vi "ni579x Host Driven Synchronization.vi"(0 "Register Buses":T1[](array[typedef]), 11 "error in":errorcluster, 12 "sync.cptr.period":u16=13) -> (4 "Register Buses (out)":T1[](array[typedef]), 15 "error out":errorcluster)   [LabVIEW 2015, in "ni579x Synchronization v2 Host.lvlib"]
doc: "Use this flavor of synchronization in conjunction with \"ni579x Host Align\" on the FPGA. Please refer to the FPGA VIs for documentation. After this VI finishes, the FPGAs will be synchronized.\n\n<B>Input Parameters</B>\n\n<B>Register Buses</B> specifies the Register Buses to which the Synchronization library is connected in the FPGA VIs.\n\n<B>sync.cptr.period</B> is the period (in clocks) of the Common Periodic Time Reference (CPTR). The CPTR period controls the rate at which synchronized signals are realized. This parameter is optional, and defaults to 13.\n\nWhen using 'ni579x FPGA Align', the CPTR period must be the same as the reference clock period. The 'sync.cptr.period' must be set to the ratio of the Single Cycle Timed Loop (SCTL) rate (that the Alignment VI is in) to the 'sync.meas.Reference Clock' rate. For example, the CPTR period must be 13 if using the PXI_Clk10 for the reference clock, and the IO Module\\Sample Clock for the SCTL clock (130 MHz / 10 MHz).\n\nWhen using 'ni579x Host Align', this value is configurable. The maximum value is 63. The minimum value for the 'sync.cptr.period' must be big enough to ensure transmission across the 'sync.cptr.FPGA I/O' line. Refer to the specifications for the FPGA I/O line chosen. For example, if the FPGA I/O line has a maximum propagation delay of 50ns, then the minimum value would be 7 (the period of the 130 MHz IO Module\\Sample Clock is ~7.692ns, so it would require 7 clocks to exceed 50ns). It is not recommended to change the CPTR period on-the-fly. Alignment must be re-run if the CPTR period is changed.\n\n<B>error in</B> describes error conditions that occur before this node runs. This input provides standard 'error in' functionality.\n\n<B>Output Parameters</B>\n\n<B>Register Buses (out)</B> passes the Register Buses to the next VI.\n\n<B>error out</B> contains error information. This output provides standard 'error out' functionality."
uses:
  <instrlib>/ni579x/Synchronization/v2/Host/ni579x Synchronization v2 Host.lvlib
  <instrlib>/_niInstr/Register Bus/v0/Host/Public/Register Bus Session.ctl
  <instrlib>/_niInstr/Register Bus/v0/Host/Private/Session Data.ctl
  <instrlib>/_niInstr/Register Bus/v0/Host/niInstr Register Bus v0 Host.lvlib
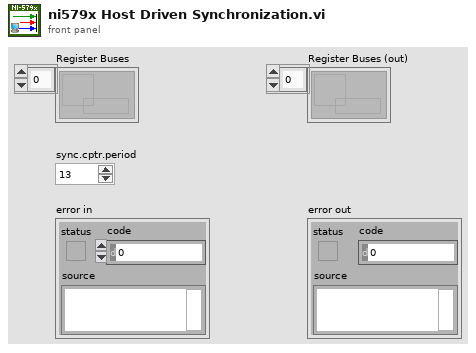
[diagram p1: front panel]
types:
  T1 = typedef "niInstr Register Bus v0 Host.lvlib/Register Bus Session.ctl" = refnum<queue>
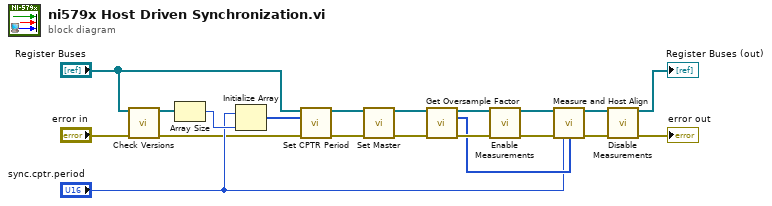
[diagram p0: block diagram]
diagram:
  n1 = call <instrlib>:"Check Versions.vi"("Register Buses"="Register Buses", "error in"="error in") -> ("Register Buses (out)"=w1:T1[], "error out"=w3:errorcluster)  [unwired: 12 in]
  n2 = Array Size(array=w1) -> (size(s)=w11:i32)
  n3 = Initialize Array("sync.cptr.period", w11) -> (w12:u16[])
  n4 = call <instrlib>:"Set CPTR Period.vi"("Register Buses"="Register Buses", "sync.cptr.period"=w12, "error in"=w3) -> ("Register Buses (out)"=w13:T1[], "error out"=w14:errorcluster)  [unwired: 11 in]
  n5 = call <instrlib>:"Set Master.vi"("Register Buses"=w13, "error in"=w14) -> ("Register Buses (out)"=w8:T1[], "error out"=w10:errorcluster)  [unwired: 12 in]
  n6 = call <instrlib>:"Get Oversample Factor.vi"("Register Buses"=w8, "error in"=w10) -> ("Register Buses (out)"=w7:T1[], "sync.meas.oversample factor"=w6:u16[], "error out"=w9:errorcluster)  [unwired: 11 in]
  n7 = call <instrlib>:"Enable Measurements.vi"("Register Buses"=w7, "error in"=w9) -> ("Register Buses (out)"=w16:T1[], "error out"=w18:errorcluster)  [unwired: 12 in]
  n8 = call <instrlib>:"Measure and Host Align.vi"("Register Buses"=w16, "error in"=w18, "sync.cptr.period"="sync.cptr.period", "sync.meas.oversample factor"=w6) -> ("Register Buses (out)"=w15:T1[], "error out"=w20:errorcluster)  [unwired: 10 in]
  n9 = call <instrlib>:"Disable Measurements.vi"("Register Buses"=w15, "error in"=w20) -> ("Register Buses (out)"=→"Register Buses (out)":T1[], "error out"=→"error out":errorcluster)  [unwired: 12 in]
